vi "MainVI.vi"() -> ()   [LabVIEW 2015]
panel:
  out "Array":dbl[](array[numeric])
  in  "stop (F)":bool
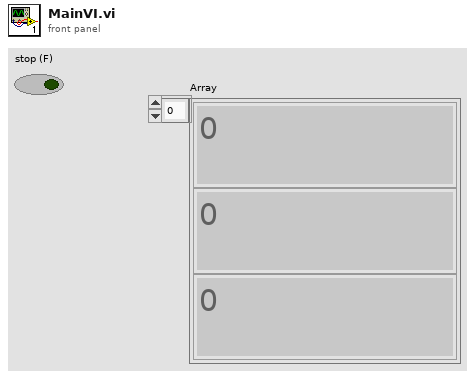
[diagram p1: front panel]
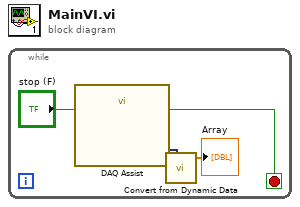
[diagram p0: block diagram]
diagram:
  n1 = while {
    stop <- w3 stop-if-true
    n2 = call "DAQ Assist.vi"("stop (F)"="stop (F)") -> ("data"=w2:dynamicdata, "stopped"=w3:bool)  [unwired: 15 in, 2 out]
    n3 = call "Convert from Dynamic Data"("Dynamic Data Type"=w2) -> ("Array"=→"Array":dbl[])  [unwired: 3 in]
  }
